vi "CalTypeToString.vi"(3 "Calibration type":T1) -> (1 "String":string)   [LabVIEW 2016]
uses:
  ADAM Client/Sub VIs/ADAM Controls/Calib_type_ADAM.ctl
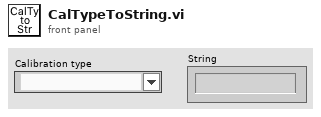
[diagram p1: front panel]
types:
  T1 = typedef "Calib_type_ADAM.ctl" = string
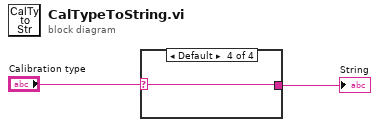
[diagram p0: block diagram]
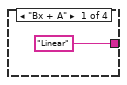
[diagram p2: hidden frame]
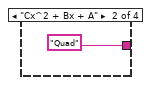
[diagram p3: hidden frame]
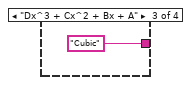
[diagram p4: hidden frame]
diagram:
  n1 = case shown="Default" "Calibration type" {
    selector: "Calibration type" -> [_ _ _ w6]
    tunnel: ["Linear" "Quad" "Cubic" w6] -> w2
    frame "Bx + A" {
    }
    frame "Cx^2 + Bx + A" {
    }
    frame "Dx^3 + Cx^2 + Bx + A" {
    }
    frame Default {
    }
  }
  "String" <- w2
